vi "Create Message-Enqueuer References VI Name.vi"() -> (0 "Create Message Enqueue References VI":string="Create Message Enqueue References.vi")   [LabVIEW 2018, in "Scripting.lvlib"]
uses:
  Scripting.lvlib
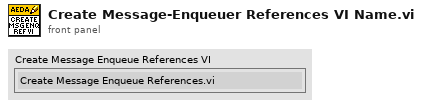
[diagram p1: front panel]
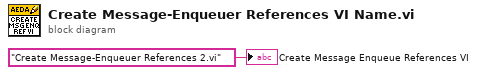
[diagram p0: block diagram]
diagram:
  "Create Message Enqueue References VI" <- "Create Message-Enqueuer References 2.vi"
